vi "Util_Convert Time Stamp to String.vi"(11 "Time":timestamp format="%<%I:%M:%S %p\n%x>T") -> (3 "Time":string)   [LabVIEW 2016]
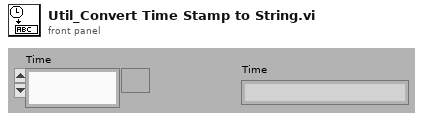
[diagram p1: front panel]
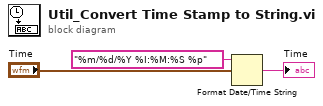
[diagram p0: block diagram]
diagram:
  n1 = Format Date/Time String(time format string (%c)="%m/%d/%Y %I:%M:%S %p", seconds (now)="Time") -> (date/time string=→"Time":string)  [unwired: 1 out]
